vi "DO Coil UI.vi"(8 "error in (no error)":errorcluster, 11 "Node Ptr":T2 format="%.0x") -> (0 "error out":errorcluster)   [LabVIEW 2021, in "Modbus Master System Explorer.lvlib"]
uses:
  Modbus Master System Explorer.lvlib
  <vilib>/NI VeriStand/Custom Device API/Custom Device Item Ref.ctl
  SubVIs/Direction.ctl
  SubVIs/Modbus Type.ctl
  <vilib>/NI VeriStand/Custom Device API/Custom Device API.lvlib
  Shared/Modbus Master Shared.lvlib
panel:
  in  "Unit ID":u8
  in  "Direction":T1
  out "Valid?":string
  in  "Address":u16
  in  "Header":cluster{"Section Name":string}={"Section Name"="Coil (Digital Out)"}
  in  "Description":string
  in  "Name":string
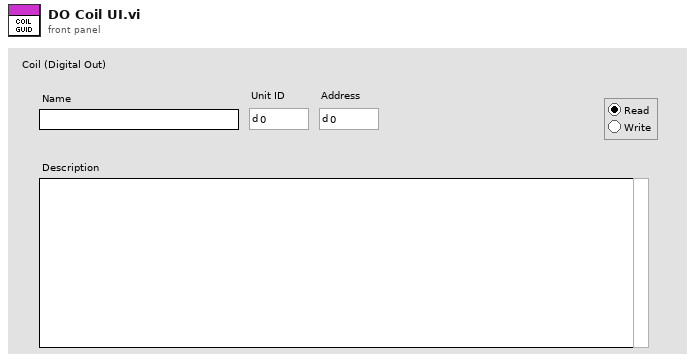
[diagram p1: front panel]
types:
  T1 = typedef "Modbus Master System Explorer.lvlib/Direction.ctl" = enum32{"Radio Selection 1", "Radio Selection 2"}
  T2 = typedef "Custom Device API.lvlib/Custom Device Item Ref.ctl" = u64
  T3 = typedef "Modbus Master Shared.lvlib/Modbus Type.ctl" = enum16{"Coil", "Discrete Input", "Holding Register", "Input Register"}
  T4 = typedef "Custom Device API.lvlib/Custom Device Commands.ctl" = enum16{"Default", "Item renamed", "Shutdown", "Dynamic button pressed"}
  T5 = typedef "Custom Device API.lvlib/Custom Device Item Info.ctl" = cluster{"Name":string, "Is Channel":bool, "GUID":string, "Is Waveform":bool}
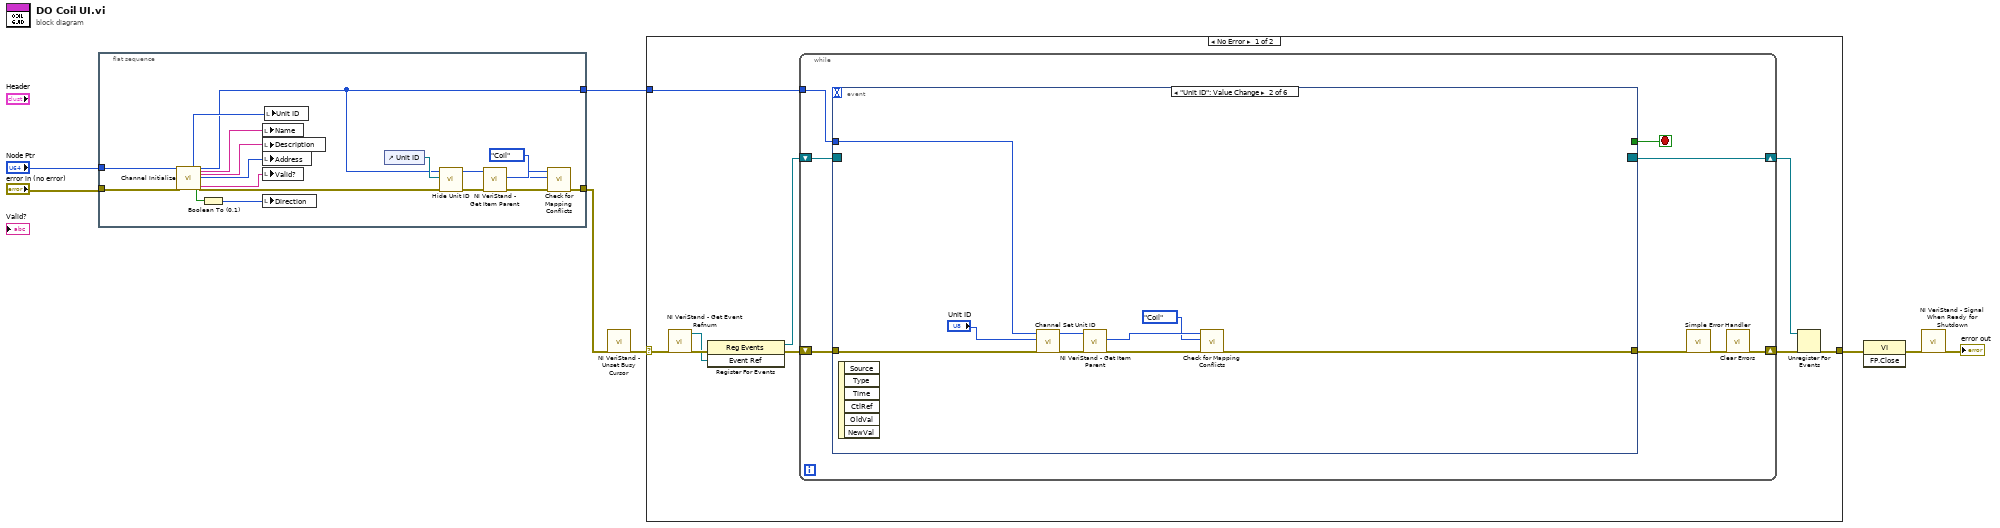
[diagram p0: block diagram]
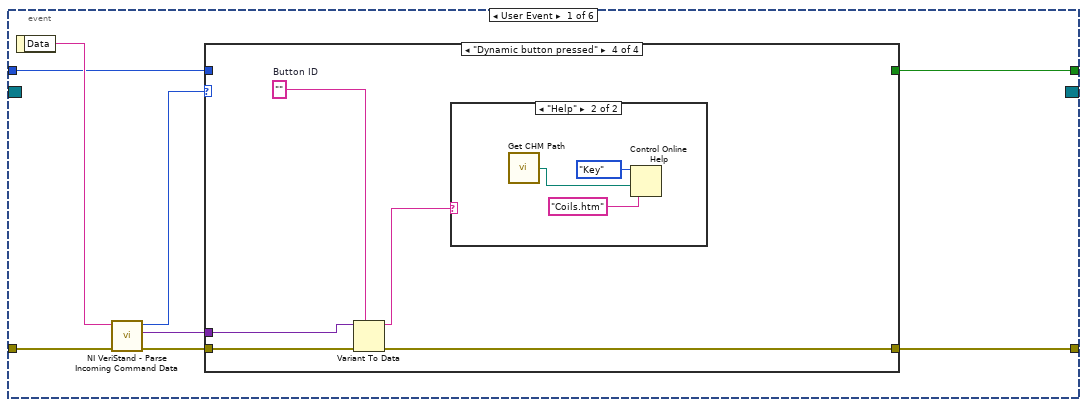
[diagram p2: hidden frame]
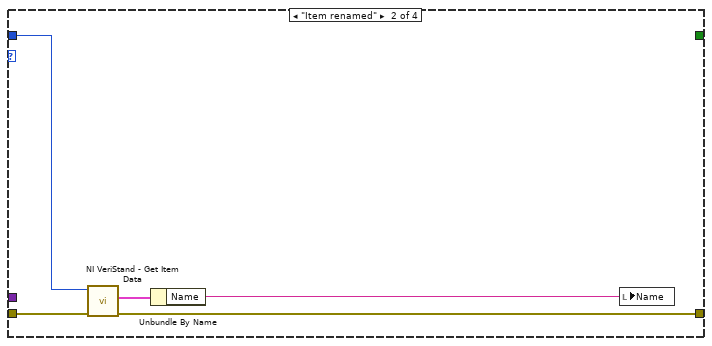
[diagram p4: hidden frame]
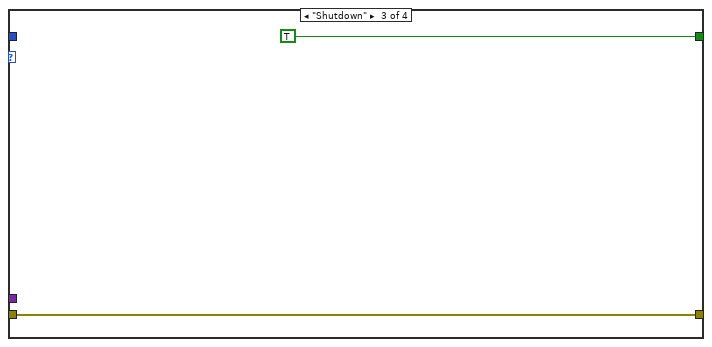
[diagram p5: hidden frame]
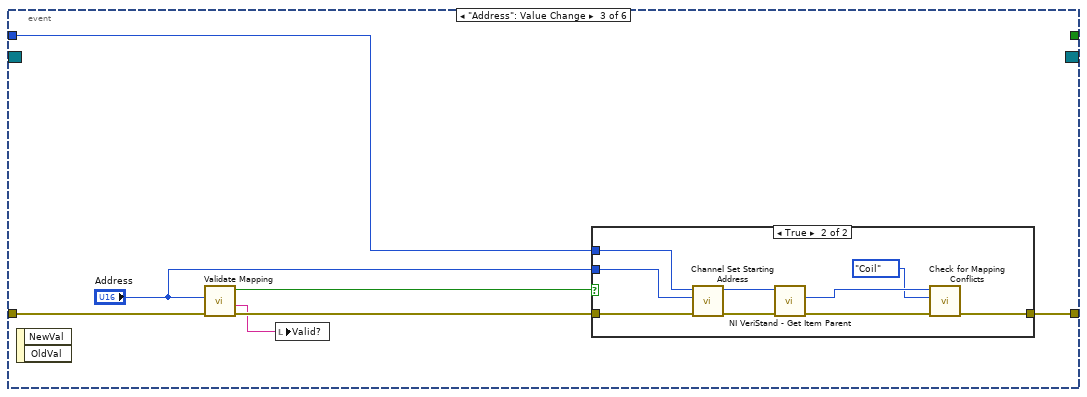
[diagram p7: hidden frame]
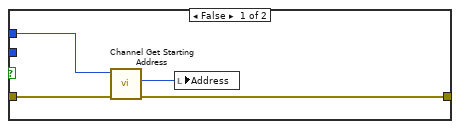
[diagram p8: hidden frame]
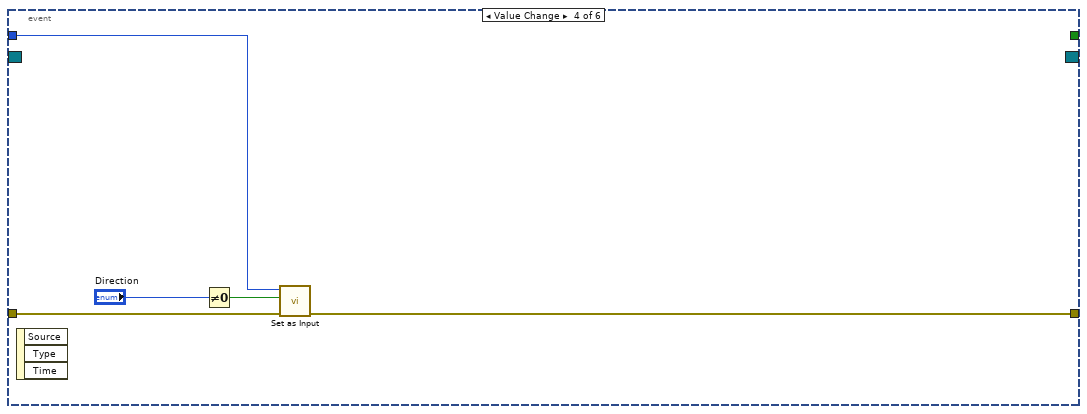
[diagram p9: hidden frame]
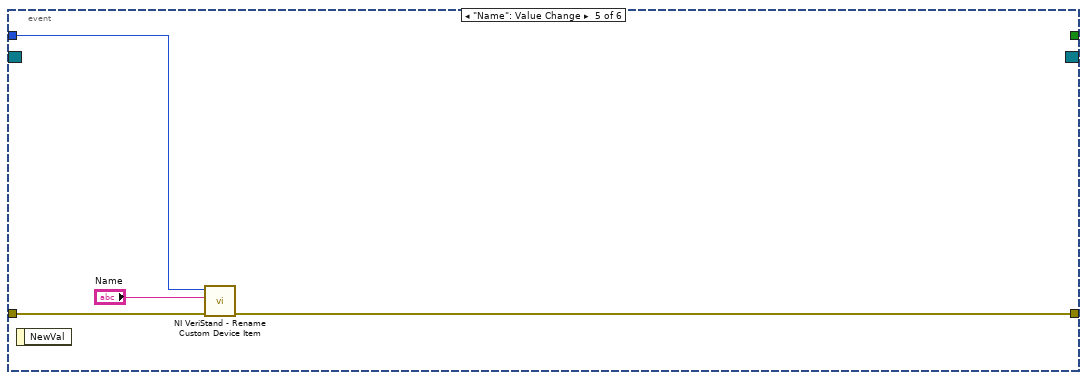
[diagram p10: hidden frame]
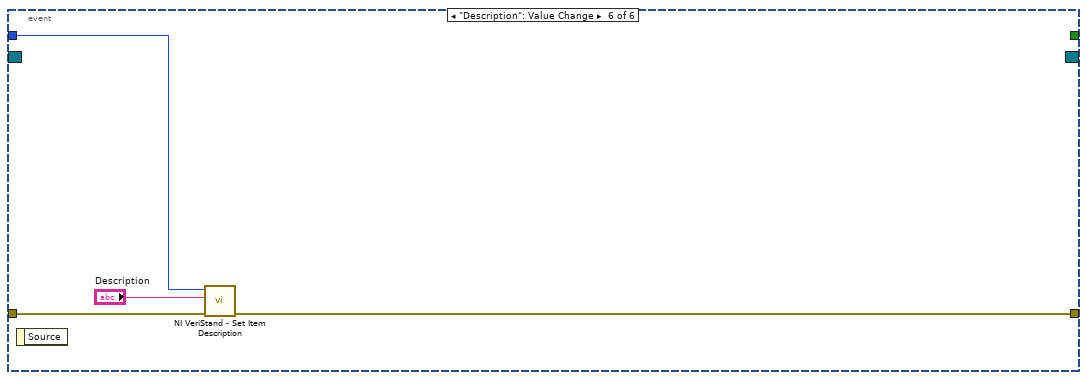
[diagram p11: hidden frame]
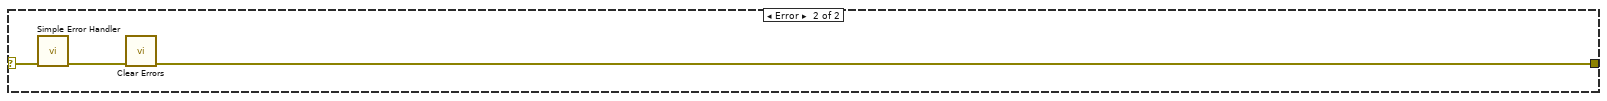
[diagram p12: hidden frame]
diagram:
  n1 = flat-sequence {
    tunnel: "Node Ptr" -> [w26]
    tunnel: [w9] -> w3
    tunnel: "error in (no error)" -> [w19]
    tunnel: [w14] -> w1
    frame #0 {
      n2 = call "Channel Initialize.vi"("Item Ref in"=w26, "error in (no error)"=w19) -> ("Unit ID"=w18:u8, "input?"=w25:bool, "Channel Ref out"=w9:T2, "Name"=w21:string, "Description"=w20:string, "Starting Address"=w22:u16, "Status Message"=w23:string, "error out"=w11:errorcluster)  [unwired: 13 in, 5 out]
      n3 = Boolean To (0,1)(Boolean=w25) -> (0, 1=w24:i16)
      n4 = local write "Name"(w21) -> ()
      n5 = local write "Description"(w20) -> ()
      n6 = local write "Address"(w22) -> ()
      n7 = local write "Valid?"(w23) -> ()
      n8 = local write "Direction"(w24) -> ()
      n9 = local write "Unit ID"(w18) -> ()
      n10 = control-ref of="Unit ID"() -> (w12:refnum<vi>)
      n11 = call "Hide Unit ID.vi"("error in (no error)"=w11, "Ctrl Ref"=w12, "Item Ref in"=w9) -> ("error out"=w10:errorcluster, "Item Ref out"=w13:T2)  [unwired: 7 in]
      n12 = call <vilib>:"NI VeriStand - Get Item Parent.vi"("error in (no error)"=w10, "Item Ref in"=w13) -> ("error out"=w15:errorcluster, "Parent Ref"=w17:T2)  [unwired: 6 in, 2 out]
      n13 = call "Check for Mapping Conflicts.vi"("error in (no error)"=w15, "Type"=Modbus_Type."Coil", "Coiil Group Ref in in"=w17) -> ("error out"=w14:errorcluster)  [unwired: 5 in, 3 out]
    }
  }
  n14 = call <vilib>:"NI VeriStand - Unset Busy Cursor.vi"("error in (no error)"=w1) -> ("error out"=w5:errorcluster)  [unwired: 10 out]
  n15 = case shown="No Error" w5 {
    selector: w5 -> [w28 w112]
    tunnel: [w32 w110] -> w8
    tunnel: w3 -> [w29 _]
    frame No Error {
      n16 = call <vilib>:"NI VeriStand - Get Event Refnum.vi"("error in (no error)"=w28) -> ("error out"=w35:errorcluster, "Event Ref"=w27:refnum<user-event>)  [unwired: 9 out]
      n17 = register-events(error in=w35, w27) -> (reference out=w30:refnum<event-registration>, error out=w31:errorcluster)  [unwired: 1 in]
      n18 = while {
        tunnel: w29 -> [w39]
        shift-right: [w36] -> w33
        shift-left: w31 -> [w42]
        shift-right: [w43] -> w34
        shift-left: w30 -> [w41]
        stop <- w40 stop-if-true
        n19 = event shown="[1] \"Unit ID\": Value Change" {
          selector: w41 -> [_ _ _ _ _ _]
          dyn-events: [_ _ _ _ _ _] -> w43
          timeout: _ -> [_ _ _ _ _ _]
          tunnel: w42 -> [w51 w75 w82 w100 w105 w108]
          tunnel: [w47 _ _ _ _ _] -> w40
          tunnel: [w46 w68 w77 w99 w104 w107] -> w38
          tunnel: w39 -> [w45 w76 w80 w101 w103 w109]
          event User Event {
            n20 = event-data() -> ("Data"=w50:string)  [unwired: 1 out]
            n21 = call <vilib>:"NI VeriStand - Parse Incoming Command Data.vi"("error in (no error)"=w51, "Incoming data"=w50) -> ("error out"=w49:errorcluster, "Outgoing data"=w44:variant, "Action"=w48:T4)  [unwired: 7 out]
            n22 = case shown="\"Dynamic button pressed\"" w48 {
              tunnel: w49 -> [w52 w57 w58 w64]
              tunnel: [_ _ TRUE _] -> w47
              tunnel: [w52 w54 w58 w61] -> w46
              tunnel: w45 -> [_ w56 _ _]
              tunnel: w44 -> [_ _ _ w63]
              frame "Default", Default {
              }
              frame "Item renamed" {
                n23 = call <vilib>:"NI VeriStand - Get Item Data.vi"("error in (no error)"=w57, "Item Ref in"=w56) -> ("error out"=w54:errorcluster, "Item Info"=w55:T5)  [unwired: 8 out]
                n24 = Unbundle By Name(w55) -> ("Name"=w53:string)
                n25 = local write "Name"(w53) -> ()
              }
              frame "Shutdown" {
              }
              frame "Dynamic button pressed" {
                w62 = ""  # Button ID
                n26 = Variant To Data(error in=w64, type=w62, Variant=w63) -> (data=w60:string, error out=w61:errorcluster)
                n27 = case shown="\"Help\"" w60 {
                  frame Default {
                  }
                  frame "Help" {
                    n28 = call "Get CHM Path.vi"() -> ("appended path"=w67:path)
                    n29 = Control Online Help(2:w67, 3:"Coils.htm" ("String to search for"), 4:enum16{"Contents", "Key", "Close"}."Key" ("Operation")) -> ()  [unwired: 1 in, 1 out]
                  }
                }
              }
            }
          }
          event "Unit ID": Value Change {
            n30 = event-data() -> ()  [unwired: 7 out]
            n31 = call "Channel Set Unit ID.vi"("error in (no error)"=w75, "Value"="Unit ID", "Item Ref in"=w76) -> ("error out"=w70:errorcluster, "Item Ref out"=w71:T2)  [unwired: 7 in]
            n32 = call <vilib>:"NI VeriStand - Get Item Parent.vi"("error in (no error)"=w70, "Item Ref in"=w71) -> ("error out"=w69:errorcluster, "Parent Ref"=w73:T2)  [unwired: 6 in, 2 out]
            n33 = call "Check for Mapping Conflicts.vi"("error in (no error)"=w69, "Type"=Modbus_Type."Coil", "Coiil Group Ref in in"=w73) -> ("error out"=w68:errorcluster)  [unwired: 5 in, 3 out]
          }
          event "Address": Value Change {
            n34 = event-data() -> ()  [unwired: 3 out]
            n35 = call "Validate Mapping.vi"("error in (no error)"=w82, "Mapping"="Address") -> ("error out"=w81:errorcluster, "Status Message"=w79:string, "Valid?"=w83:bool)  [unwired: 7 in]
            n36 = local write "Valid?"(w79) -> ()
            n37 = case shown="True" w83 {
              tunnel: w81 -> [w87 w94]
              tunnel: w80 -> [w84 w96]
              tunnel: "Address" -> [_ w95]
              tunnel: [w86 w89] -> w77
              frame False {
                n38 = call "Channel Get Starting Address.vi"("error in (no error)"=w87, "Item Ref in"=w84) -> ("error out"=w86:errorcluster, "Value"=w85:u16)  [unwired: 7 in, 1 out]
                n39 = local write "Address"(w85) -> ()
              }
              frame True {
                n40 = call "Channel Set Starting Address.vi"("error in (no error)"=w94, "Value"=w95, "Item Ref in"=w96) -> ("error out"=w91:errorcluster, "Item Ref out"=w93:T2)  [unwired: 7 in]
                n41 = call <vilib>:"NI VeriStand - Get Item Parent.vi"("error in (no error)"=w91, "Item Ref in"=w93) -> ("error out"=w90:errorcluster, "Parent Ref"=w92:T2)  [unwired: 6 in, 2 out]
                n42 = call "Check for Mapping Conflicts.vi"("error in (no error)"=w90, "Type"=Modbus_Type."Coil", "Coiil Group Ref in in"=w92) -> ("error out"=w89:errorcluster)  [unwired: 5 in, 3 out]
              }
            }
          }
          event Value Change {
            n43 = event-data() -> ()  [unwired: 4 out]
            n44 = Not Equal To 0?(x="Direction") -> (x != 0?=w97:bool)
            n45 = call "Set as Input.vi"("error in (no error)"=w100, "Direction"=w97, "Channel Ref in"=w101) -> ("error out"=w99:errorcluster)  [unwired: 7 in, 1 out]
          }
          event "Name": Value Change {
            n46 = event-data() -> ()  [unwired: 2 out]
            n47 = call <vilib>:"NI VeriStand - Rename Custom Device Item.vi"("error in (no error)"=w105, "New Name"="Name", "Item Ref in"=w103) -> ("error out"=w104:errorcluster)  [unwired: 1 in, 7 out]
          }
          event "Description": Value Change {
            n48 = event-data() -> ()  [unwired: 2 out]
            n49 = call <vilib>:"NI VeriStand - Set Item Description.vi"("error in (no error)"=w108, "Description"="Description", "Item Ref in"=w109) -> ("error out"=w107:errorcluster)  [unwired: 8 out]
          }
        }
        n50 = call <vilib>:"Simple Error Handler.vi"("error in (no error)"=w38) -> ("error out"=w37:errorcluster)  [unwired: 1 in, 7 out]
        n51 = call <vilib>:"Clear Errors.vi"("error in (no error)"=w37) -> ("error out"=w36:errorcluster)  [unwired: 1 in, 5 out]
      }
      n52 = Unregister For Events(event registration refnum=w34, error in=w33) -> (error out=w32:errorcluster)
    }
    frame Error {
      n53 = call <vilib>:"Simple Error Handler.vi"("error in (no error)"=w112) -> ("error out"=w111:errorcluster)  [unwired: 1 in, 7 out]
      n54 = call <vilib>:"Clear Errors.vi"("error in (no error)"=w111) -> ("error out"=w110:errorcluster)  [unwired: 1 in, 5 out]
    }
  }
  n55 = invoke class="VI" method="FP.Close"(error in=w8) -> (error out=w7:errorcluster)  [unwired: 2 in, 2 out]
  n56 = call <vilib>:"NI VeriStand - Signal When Ready for Shutdown.vi"("error in (no error)"=w7) -> ("error out"=→"error out":errorcluster)  [unwired: 10 out]
